vi "Timer LED Sequence.vi"(11 "Reverse?":bool) -> (0 "LED3":bool, 1 "LED2":bool, 2 "LED1":bool, 3 "LED0":bool)   [LabVIEW 2021]
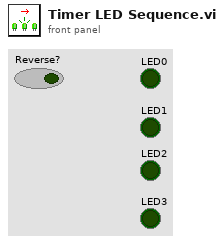
[diagram p1: front panel]
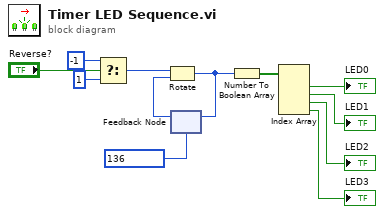
[diagram p0: block diagram]
diagram:
  n1 = Select(t=i8 -1 ("f"), s="Reverse?", f=i8 1 ("y")) -> (s? t:f=w3:i8)
  n2 = feedback #1(u8 136) -> (w7:u8)
  n3 = Rotate(1:w7, 2:w3) -> (0:w6:u8)
  n4 = feedback-in #1(w6) -> ()
  n5 = Number To Boolean Array(number=w6) -> (Boolean array=w12:bool[])
  n6 = Index Array(array=w12) -> (element #1=→"LED0":bool, element #2=→"LED1":bool, element #3=→"LED2":bool, element #4=→"LED3":bool)  [unwired: 4 in]
